vi "Open Selected VI Location.vi"(6 "Variant in":variant, 7 "Shift Pressed?":bool, 8 "error in (no error)":errorcluster, 10 "QD Combo Box Ref":refnum<vi>, 11 "QD Launch VI Ref":refnum<vi>) -> (0 "error out":errorcluster, 4 "Variant out":variant)   [LabVIEW 2012, in "Smart Open VI Location.lvlib"]
doc: "Open Selected VI's Location in Explorer Window."
uses:
  Smart Open VI Location.lvlib
  <userlib>/_OpenG.lib/file/file.llb/Valid Path - Traditional__ogtk.vi
panel:
  in  "Undo Name":string="Quick Drop Keyboard Shortcut"
  # "Do not change the connector pane of this VI.\n\nSee the block diagram for directions on how to use this template."
  # "Specify the name of the Undo transaction"
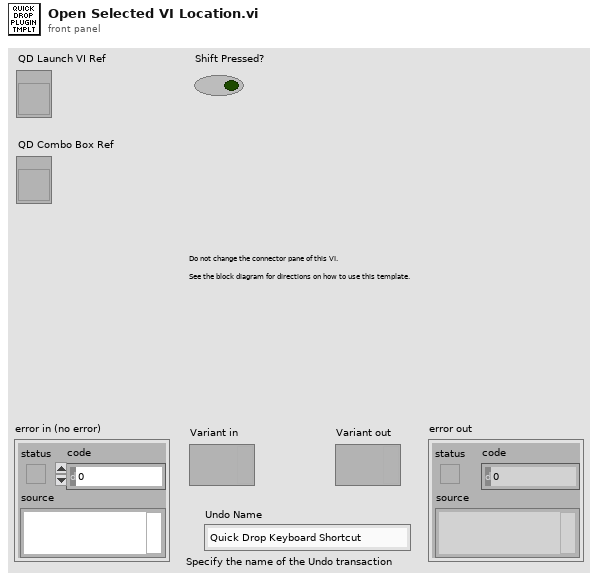
[diagram p1: front panel]
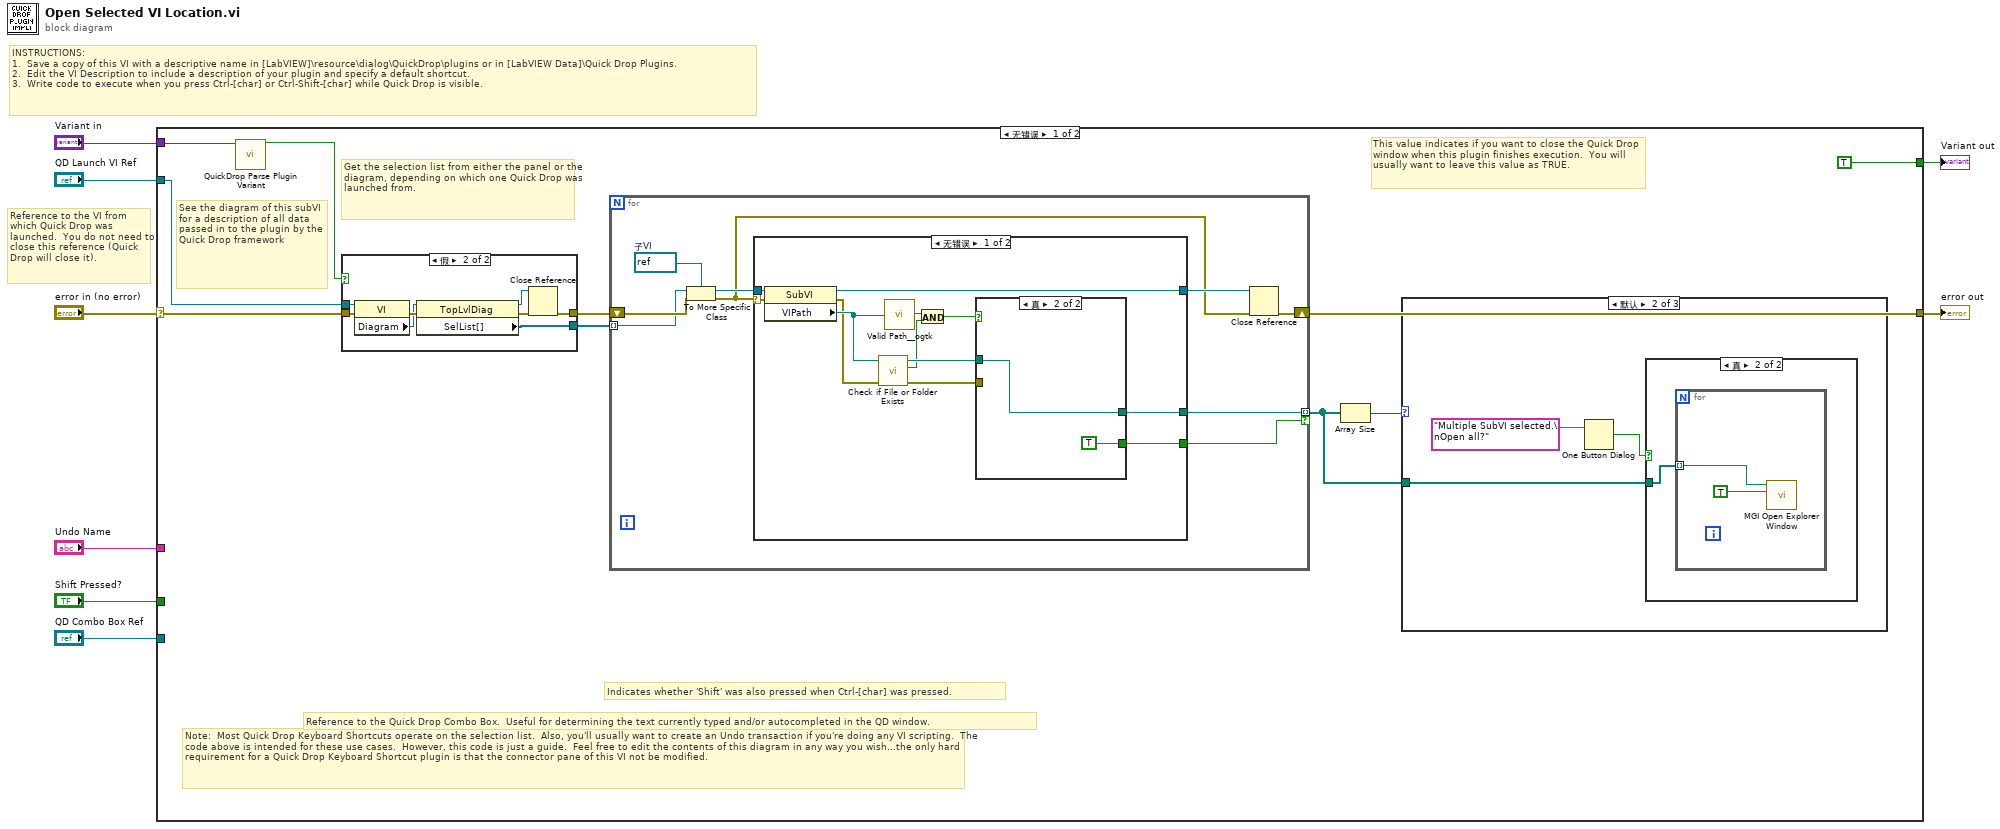
[diagram p0: block diagram]
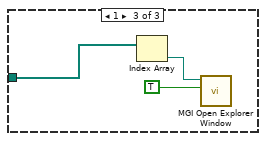
[diagram p4: hidden frame]
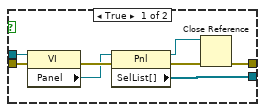
[diagram p7: hidden frame]
diagram:
  # "Reference to the VI from which Quick Drop was launched.  You do not need to close this reference (Quick Drop will close it)."
  # "INSTRUCTIONS:\n1.  Save a copy of this VI with a descriptive name in [LabVIEW]\\resource\\dialog\\QuickDrop\\plugins or in [LabVIEW Data]\\Quick Drop Plugins.\n2.  Edit the VI Description to include a description of your plugin and specify a default shortcut. \n3.  Write code to execute when you press Ctrl-[char] or Ctrl-Shift-[char] while Quick Drop is visible."
  n1 = case shown="无错误" "error in (no error)" {
    selector: "error in (no error)" -> [w17 w68]
    tunnel: [w11 w68] -> w7
    tunnel: "QD Launch VI Ref" -> [w16 _]
    tunnel: "Shift Pressed?" -> [_ _]
    tunnel: "QD Combo Box Ref" -> [_ _]
    tunnel: "Variant in" -> [w18 _]
    tunnel: "Undo Name" -> [_ _]
    tunnel: [TRUE _] -> w1
    frame No Error {
      # "Note:  Most Quick Drop Keyboard Shortcuts operate on the selection list.  Also, you'll usually want to create an Undo transaction if you're doing any VI scripting.  The code above is intended for these use cases.  However, this code is just a guide.  Feel free to edit the contents of this diagram in any way you wish...the only hard requirement for a Quick Drop Keyboard Shortcut plugin is that the connector pane of this VI not be modified."
      # "Get the selection list from either the panel or the diagram, depending on which one Quick Drop was launched from."
      # "This value indicates if you want to close the Quick Drop window when this plugin finishes execution.  You will usually want to leave this value as TRUE."
      # "See the diagram of this subVI for a description of all data passed in to the plugin by the Quick Drop framework"
      # "Reference to the Quick Drop Combo Box.  Useful for determining the text currently typed and/or autocompleted in the QD window."
      # "Indicates whether 'Shift' was also pressed when Ctrl-[char] was pressed."
      n2 = call <vilib>:"QuickDrop Parse Plugin Variant.vi"("QDKS Variant in"=w18) -> ("QD Launch VI Panel?"=w14:bool)  [unwired: 12 in, 2 out]
      n3 = case shown="假" w14 {
        tunnel: w17 -> [w59 w67]
        tunnel: w16 -> [w58 w66]
        tunnel: [w53 w61] -> w13
        tunnel: [w52 w60] -> w12
        frame True {
          n4 = property class="VI"(reference=w58, error in=w59) -> (error out=w57:errorcluster, "Panel"=w56:refnum<vi>)  [unwired: 1 out]
          n5 = property class="Pnl"(reference=w56, error in=w57) -> (reference out=w54:refnum<vi>, error out=w55:errorcluster, "SelList[]"=w52:refnum<vi>[])
          n6 = Close Reference(reference=w54, error in (no error)=w55) -> (error out=w53:errorcluster)
        }
        frame False {
          n7 = property class="VI"(reference=w66, error in=w67) -> (error out=w65:errorcluster, "Diagram"=w64:refnum<vi>)  [unwired: 1 out]
          n8 = property class="TopLvlDiag"(reference=w64, error in=w65) -> (reference out=w62:refnum<vi>, error out=w63:errorcluster, "SelList[]"=w60:refnum<vi>[])
          n9 = Close Reference(reference=w62, error in (no error)=w63) -> (error out=w61:errorcluster)
        }
      }
      n10 = for {
        shift-right: [w36] -> w11
        shift-left: w13 -> [w34]
        tunnel: w12 -> [w33] mode=indexing
        tunnel: [w29] -> w9 mode=indexing if=w28
        w30 = refnum<vi> refnum  # 子VI
        n11 = To More Specific Class(target class=w30, reference=w33, error in=w34) -> (specific class reference=w32:refnum<vi>, error out=w31:errorcluster)
        n12 = case shown="无错误" w31 {
          selector: w31 -> [w47 _]
          tunnel: [w48 w51] -> w35
          tunnel: w32 -> [w46 w51]
          tunnel: [w38 _] -> w29
          tunnel: [w37 _] -> w28
          frame No Error {
            n13 = property class="SubVI"(reference=w46, error in=w47) -> (reference out=w48:refnum<vi>, error out=w39:errorcluster, "VIPath"=w40:path)
            n14 = call <vilib>:"Check if File or Folder Exists.vi"("error in (no error)"=w39, "path"=w40) -> ("error out"=w44:errorcluster, "file or folder exists?"=w42:bool, "dup path"=w45:path)  [unwired: 7 in]
            n15 = call-poly <userlib>:"Valid Path__ogtk.vi"("path"=w40) -> ("valid"=w43:bool)
            n16 = And(x=w43, y=w42) -> (x .and. y?=w41:bool)
            n17 = case shown="真" w41 {
              tunnel: w45 -> [_ w50]
              tunnel: w44 -> [_ _]
              tunnel: [_ w50] -> w38
              tunnel: [_ TRUE] -> w37
              frame False {
              }
              frame True {
              }
            }
          }
          frame Error {
          }
        }
        n18 = Close Reference(reference=w35, error in (no error)=w31) -> (error out=w36:errorcluster)
      }
      n19 = Array Size(array=w9) -> (size(s)=w10:i32)
      n20 = case shown="默认" w10 {
        tunnel: w9 -> [_ w20 w26]
        frame 0 {
        }
        frame Default {
          n21 = One Button Dialog(message="Multiple SubVI selected.\nOpen all?") -> (true=w19:bool)  [unwired: 1 in]
          n22 = case shown="真" w19 {
            tunnel: w20 -> [_ w22]
            frame False {
            }
            frame True {
              n23 = for {
                tunnel: w22 -> [w23] mode=indexing
                n24 = call <userlib>:"MGI Open Explorer Window.vi"("Select Directory? (F: Open Directory)"=TRUE, "Directory or File"=w23) -> ()  [unwired: 9 in, 1 out]
              }
            }
          }
        }
        frame 1 {
          n25 = Index Array(array=w26) -> (element=w25:path)  [unwired: 1 in]
          n26 = call <userlib>:"MGI Open Explorer Window.vi"("Select Directory? (F: Open Directory)"=TRUE, "Directory or File"=w25) -> ()  [unwired: 9 in, 1 out]
        }
      }
    }
    frame Error {
    }
  }
  "error out" <- w7
  "Variant out" <- w1
